vi "ExSubDisplaySaveMultiFrame.vi"(0 "Number of Images":u32, 1 "Display Handle":u32, 2 "file handle":u32, 3 "error in (no error)":errorcluster, 4 "Data handles":u32[](array[numeric])) -> (5 "Display Handle":u32, 6 "file Handle":u32, 7 "error out":errorcluster)   [LabVIEW 2010]
panel:
  # "ExSubDisplaySaveMultiFrame.vi\nThis sub VI takes an array of image handles and pulls them out of \narray, displays the image then stores the image in file.\nUser may want to put a delay in loop so he sees the images as they \nare displayed or remove the display part for a real application."
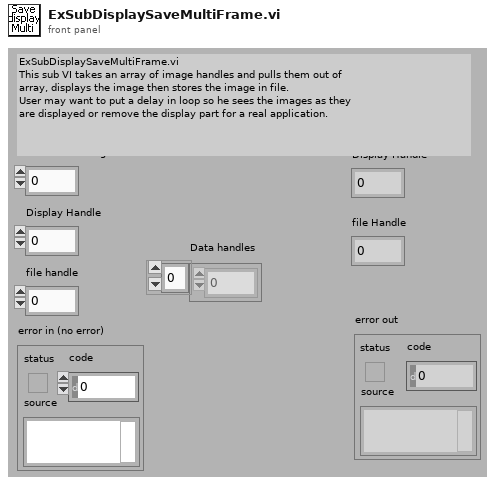
[diagram p1: front panel]
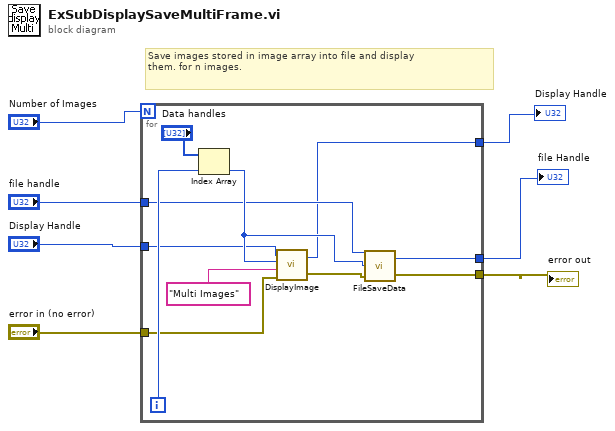
[diagram p0: block diagram]
diagram:
  # "Save images stored in image array into file and display\nthem. for n images."
  n1 = for {
    N: "Number of Images" -> [_]
    tunnel: "Display Handle" -> [w15]
    tunnel: "file handle" -> [w14]
    tunnel: "error in (no error)" -> [w12]
    tunnel: [w11] -> w3
    tunnel: [w9] -> w2
    tunnel: [w8] -> w1
    i -> [w18]
    n2 = Index Array(array="Data handles", index=w18) -> (element=w16:u32)
    n3 = call <userlib>:"DisplayImage.vi"("error in"=w12, "Title"="Multi Images", "Image Handle"=w16, "Display Handle"=w15) -> ("error out"=w13:errorcluster, "Display Handle"=w8:u32)
    n4 = call <userlib>:"FileSaveData.vi"("error in"=w13, "Image Handle"=w16, "File Handle"=w14) -> ("error out"=w11:errorcluster, "File Handle"=w9:u32)
  }
  "error out" <- w3
  "file Handle" <- w2
  "Display Handle" <- w1
